vi "RSZVB Set Fixed Power.vi"(8 "error in (no error)":errorcluster {"code" format="%.0x"}, 9 "Fixed Power (-25.0)":dbl=-25.0 format="%^.3e", 10 "Channel (1)":i32=1, 11 "VISA session":refnum<visa-resource-name>) -> (0 "error out":errorcluster {"code" format="%.0x"}, 3 "dup VISA session":refnum<visa-resource-name>)   [LabVIEW 2011]
doc: "This VI defines a fixed power, to be assigned either to the RF or to the LO signal.\n\nRemote-control command(s):\nSOURce<Ch>:FREQuency:CONVersion:MIXer:PFIXed <fixed_power>"
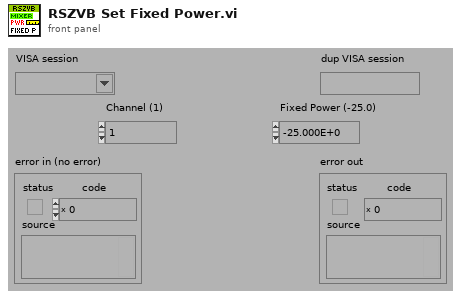
[diagram p1: front panel]
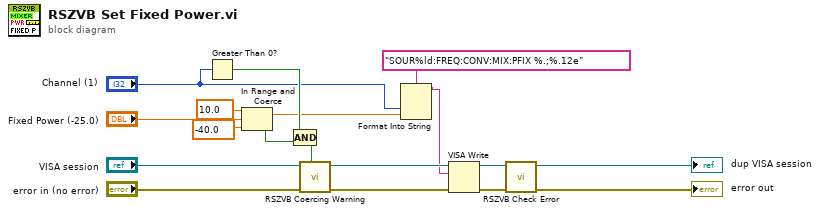
[diagram p0: block diagram]
diagram:
  n1 = Greater Than 0?(x="Channel (1)") -> (x > 0?=w13:bool)
  n2 = In Range and Coerce(upper limit=10.0, x="Fixed Power (-25.0)", lower limit=-40.0) -> (coerced(x)=w1:dbl, In Range?=w14:bool)
  n3 = Compound Arithmetic op=AND(w13, w14) -> (w12:bool)
  n4 = call "RSZVB Coercing Warning.vi"("In Range?"=w12, "error in (no error)"="error in (no error)", "VISA session"="VISA session") -> ("error out"=w17:errorcluster, "dup VISA session"=w18:refnum<visa-resource-name>)  [unwired: 7 in]
  n5 = Format Into String(format string="SOUR%ld:FREQ:CONV:MIX:PFIX %.;%.12e", "Channel (1)", w1) -> (resulting string=w2:string)  [unwired: 2 in, 1 out]
  n6 = VISA Write(VISA resource name=w18, write buffer=w2, error in (no error)=w17) -> (VISA resource name out=w15:refnum<visa-resource-name>, error out=w16:errorcluster)  [unwired: 1 out]
  n7 = call "RSZVB Check Error.vi"("error in (no error)"=w16, "VISA session"=w15) -> ("error out"=→"error out":errorcluster, "dup VISA session"=→"dup VISA session":refnum<visa-resource-name>)  [unwired: 8 in]
